vi "FeedbackDecode_FPPNS2NIP.vi"(5 "NIPTime":dbl=37572.0, 6 "EncodeClust":T2={"ParamsTable"=[], "Sel"=[], "Stim"=FALSE, "StimMode"=enum."Off", "StimStep"=[enum."1uA", enum."1uA", enum."Off"], "Jitter"=FALSE, "Pulse"=FALSE, "BFreq"=0.0, "BAmp"=0.0, "UEAArray"=[], "AdjClust"={"Add"=FALSE, "Sub"=FALSE, "Val"=[1.0, 100.0, 0.2, 500.0, 0.0], "B"=[FALSE, FALSE, FALSE, FALSE, FALSE], "Inc+"=["x+1", "x+10", "x+0.1", "x+10", "x+10"], "Set"=FALSE, "LoadTable"=FALSE, "SaveTable"=FALSE, "ClearTable"=FALSE, "DeleteSel"=FALSE, "Inc-"=["x-1", "x-10", "x-0.1", "x-10", "x-10"]}, "PresetTable"=[], "SelPreset"=[], "SortClust"={"Region"=FALSE, "Receptor"=FALSE, "Electrode"=FALSE, "Min Amp"=FALSE, "Max Amp"=FALSE, "Min Freq"=FALSE, "Max Freq"=FALSE, "Duration"=FALSE}, "SelSort"={"Sel"=FALSE}, "PresetClust"={"Load"=FALSE, "Clear"=FALSE, "Save"=FALSE, "Del"=FALSE}, "RespClust"={"RespType"=enum."Sensor Map", "OpenResp"=FALSE}, "AmpLimit"=0.0, "FreqLimit"=0.0, "DurLimit"=0.0, "Wait Period"=0.0, "Train Period"=0.0} {"Train Period" min=0.0 max=100.0 step=0.1; "Wait Period" min=0.0 max=100.0 step=0.1; "DurLimit" min=0.0 max=1.0 step=0.01; "FreqLimit" min=0.0 max=500.0 step=1.0; "AmpLimit" min=0.0 max=100.0 step=1.0; "BAmp" min=0.0 max=100.0 step=1.0; "BFreq" min=0.0 max=100.0 step=1.0}, 7 "LoopCnt":dbl=37572.0, 8 "DecodeClust":T3={"TrainParams"={"Lag"=0.0, "KernelWidth"=0.3, "TargRad"=0.15}, "Kinematics"={"Thumb"=0.0, "Index"=0.0, "Middle"=0.0, "Ring"=0.0, "Little"=0.0, "ThumbInt"=0.0, "IndexInt"=0.0, "RingInt"=0.0, "LittleInt"=0.0, "Wrist"=0.0, "WristYaw"=0.0, "WristRoll"=0.0}, "CtrlButtons"={"AcqTraining"=FALSE, "ApplyBaseline"=FALSE, "ApplyTraining"=FALSE, "LoadTrainFile"=FALSE, "CAR"=FALSE, "NIPSpikes"=FALSE, "AcqBaseline"=FALSE, "Stop"=FALSE, "ResetTrial"=FALSE, "CalDEKA"=FALSE, "HideSphrs"=FALSE, "StartTrials"=FALSE, "AutoPop"=FALSE, "ResetVRE"=FALSE, "StopVRE"=FALSE, "AcqCAR"=FALSE, "ConARD"=FALSE, "DEKARestart"=FALSE, "ConnDEKA"=FALSE}, "CompID"={"LV"={"Name"="PNILABVIEW", "IP"="155.100.90.215"}, "ML"={"Name"="PNIMATLAB", "IP"="155.100.91.231"}}, "KMvntClust"={"KGain"=[[1.0, 1.0, -1.0, 1.0], [1.0, 1.0, -1.0, 1.0], [1.0, 1.0, -1.0, 1.0], [1.0, 1.0, -1.0, 1.0], [1.0, 1.0, -1.0, 1.0], [1.0, 1.0, -1.0, 1.0], [1.0, 1.0, -1.0, 1.0], [1.0, 1.0, -1.0, 1.0], [1.0, 1.0, -1.0, 1.0], [1.0, 1.0, -1.0, 1.0], [1.0, 1.0, -1.0, 1.0], [1.0, 1.0, -1.0, 1.0]], "KMvnts"={"Thumb"=FALSE, "Index"=FALSE, "Middle"=FALSE, "Ring"=FALSE, "Little"=FALSE, "ThumbInt"=FALSE, "IndexInt"=FALSE, "RingInt"=FALSE, "LittleInt"=FALSE, "WristPitch"=FALSE, "WristYaw"=FALSE, "WristRoll"=FALSE}, "KThresh"=[[0.2, 0.2, -1.0, 1.0], [0.2, 0.2, -1.0, 1.0], [0.2, 0.2, -1.0, 1.0], [0.2, 0.2, -1.0, 1.0], [0.2, 0.2, -1.0, 1.0], [0.2, 0.2, -1.0, 1.0], [0.2, 0.2, -1.0, 1.0], [0.2, 0.2, -1.0, 1.0], [0.2, 0.2, -1.0, 1.0], [0.2, 0.2, -1.0, 1.0], [0.2, 0.2, -1.0, 1.0], [0.2, 0.2, -1.0, 1.0]], "CtrlMode"=[], "CtrlSpd"=[]}, "ClearUEA"=FALSE, "Targets"={"Thumb"=0.0, "Index"=0.0, "Middle"=0.0, "Ring"=0.0, "Little"=0.0, "ThumbInt"=0.0, "IndexInt"=0.0, "RingInt"=0.0, "LittleInt"=0.0, "Wrist"=0.0, "WristYaw"=0.0, "WristRoll"=0.0}, "KUEAArray"=[{"Boolean 1"=FALSE, "Boolean 2"=FALSE, "Boolean 3"=FALSE, "Boolean 4"=FALSE, "Boolean 5"=FALSE, "Boolean 6"=FALSE, "Boolean 7"=FALSE, "Boolean 8"=FALSE, "Boolean 9"=FALSE, "Boolean 10"=FALSE, "Boolean 11"=FALSE, "Boolean 12"=FALSE, "Boolean 13"=FALSE, "Boolean 14"=FALSE, "Boolean 15"=FALSE, "Boolean 16"=FALSE, "Boolean 17"=FALSE, "Boolean 18"=FALSE, "Boolean 19"=FALSE, "Boolean 20"=FALSE, "Boolean 21"=FALSE, "Boolean 22"=FALSE, "Boolean 23"=FALSE, "Boolean 24"=FALSE, "Boolean 25"=FALSE, "Boolean 26"=FALSE, "Boolean 27"=FALSE, "Boolean 28"=FALSE, "Boolean 29"=FALSE, "Boolean 30"=FALSE, "Boolean 31"=FALSE, "Boolean 32"=FALSE, "Boolean 33"=FALSE, "Boolean 34"=FALSE, "Boolean 35"=FALSE, "Boolean 36"=FALSE, "Boolean 37"=FALSE, "Boolean 38"=FALSE, "Boolean 39"=FALSE, "Boolean 40"=FALSE, "Boolean 41"=FALSE, "Boolean 42"=FALSE, "Boolean 43"=FALSE, "Boolean 44"=FALSE, "Boolean 45"=FALSE, "Boolean 46"=FALSE, "Boolean 47"=FALSE, "Boolean 48"=FALSE, "Boolean 49"=FALSE, "Boolean 50"=FALSE, "Boolean 51"=FALSE, "Boolean 52"=FALSE, "Boolean 53"=FALSE, "Boolean 54"=FALSE, "Boolean 55"=FALSE, "Boolean 56"=FALSE, "Boolean 57"=FALSE, "Boolean 58"=FALSE, "Boolean 59"=FALSE, "Boolean 60"=FALSE, "Boolean 61"=FALSE, "Boolean 62"=FALSE, "Boolean 63"=FALSE, "Boolean 64"=FALSE, "Boolean 65"=FALSE, "Boolean 66"=FALSE, "Boolean 67"=FALSE, "Boolean 68"=FALSE, "Boolean 69"=FALSE, "Boolean 70"=FALSE, "Boolean 71"=FALSE, "Boolean 72"=FALSE, "Boolean 73"=FALSE, "Boolean 74"=FALSE, "Boolean 75"=FALSE, "Boolean 76"=FALSE, "Boolean 77"=FALSE, "Boolean 78"=FALSE, "Boolean 79"=FALSE, "Boolean 80"=FALSE, "Boolean 81"=FALSE, "Boolean 82"=FALSE, "Boolean 83"=FALSE, "Boolean 84"=FALSE, "Boolean 85"=FALSE, "Boolean 86"=FALSE, "Boolean 87"=FALSE, "Boolean 88"=FALSE, "Boolean 89"=FALSE, "Boolean 90"=FALSE, "Boolean 91"=FALSE, "Boolean 92"=FALSE, "Boolean 93"=FALSE, "Boolean 94"=FALSE, "Boolean 95"=FALSE, "Boolean 96"=FALSE, "Boolean 97"=FALSE, "Boolean 98"=FALSE, "Boolean 99"=FALSE, "Boolean 100"=FALSE}, {"Boolean 1"=FALSE, "Boolean 2"=FALSE, "Boolean 3"=FALSE, "Boolean 4"=FALSE, "Boolean 5"=FALSE, "Boolean 6"=FALSE, "Boolean 7"=FALSE, "Boolean 8"=FALSE, "Boolean 9"=FALSE, "Boolean 10"=FALSE, "Boolean 11"=FALSE, "Boolean 12"=FALSE, "Boolean 13"=FALSE, "Boolean 14"=FALSE, "Boolean 15"=FALSE, "Boolean 16"=FALSE, "Boolean 17"=FALSE, "Boolean 18"=FALSE, "Boolean 19"=FALSE, "Boolean 20"=FALSE, "Boolean 21"=FALSE, "Boolean 22"=FALSE, "Boolean 23"=FALSE, "Boolean 24"=FALSE, "Boolean 25"=FALSE, "Boolean 26"=FALSE, "Boolean 27"=FALSE, "Boolean 28"=FALSE, "Boolean 29"=FALSE, "Boolean 30"=FALSE, "Boolean 31"=FALSE, "Boolean 32"=FALSE, "Boolean 33"=FALSE, "Boolean 34"=FALSE, "Boolean 35"=FALSE, "Boolean 36"=FALSE, "Boolean 37"=FALSE, "Boolean 38"=FALSE, "Boolean 39"=FALSE, "Boolean 40"=FALSE, "Boolean 41"=FALSE, "Boolean 42"=FALSE, "Boolean 43"=FALSE, "Boolean 44"=FALSE, "Boolean 45"=FALSE, "Boolean 46"=FALSE, "Boolean 47"=FALSE, "Boolean 48"=FALSE, "Boolean 49"=FALSE, "Boolean 50"=FALSE, "Boolean 51"=FALSE, "Boolean 52"=FALSE, "Boolean 53"=FALSE, "Boolean 54"=FALSE, "Boolean 55"=FALSE, "Boolean 56"=FALSE, "Boolean 57"=FALSE, "Boolean 58"=FALSE, "Boolean 59"=FALSE, "Boolean 60"=FALSE, "Boolean 61"=FALSE, "Boolean 62"=FALSE, "Boolean 63"=FALSE, "Boolean 64"=FALSE, "Boolean 65"=FALSE, "Boolean 66"=FALSE, "Boolean 67"=FALSE, "Boolean 68"=FALSE, "Boolean 69"=FALSE, "Boolean 70"=FALSE, "Boolean 71"=FALSE, "Boolean 72"=FALSE, "Boolean 73"=FALSE, "Boolean 74"=FALSE, "Boolean 75"=FALSE, "Boolean 76"=FALSE, "Boolean 77"=FALSE, "Boolean 78"=FALSE, "Boolean 79"=FALSE, "Boolean 80"=FALSE, "Boolean 81"=FALSE, "Boolean 82"=FALSE, "Boolean 83"=FALSE, "Boolean 84"=FALSE, "Boolean 85"=FALSE, "Boolean 86"=FALSE, "Boolean 87"=FALSE, "Boolean 88"=FALSE, "Boolean 89"=FALSE, "Boolean 90"=FALSE, "Boolean 91"=FALSE, "Boolean 92"=FALSE, "Boolean 93"=FALSE, "Boolean 94"=FALSE, "Boolean 95"=FALSE, "Boolean 96"=FALSE, "Boolean 97"=FALSE, "Boolean 98"=FALSE, "Boolean 99"=FALSE, "Boolean 100"=FALSE}], "ReTrain"=FALSE, "TargDist"=[0.0, 0.0, 0.0, 0.0, 0.0, 0.0], "State"=enum."Initialize", "KalmanType"=enum."Standard", "EventStr"="", "SelElect"=1.0, "KinSrc"=enum."Training", "HoverElect"=0.0, "RasterWin"=1.0, "WfCnt"=15.0, "ClearWfs"=FALSE, "ApplyThresh"=FALSE, "ThreshVal"=-5.0, "ThreshMode"=enum."RMS Single", "DataFolder"="00000000-000000", "ClearEMG"=FALSE, "KEMGClust"={"Boolean 92"=FALSE, "Boolean 82"=FALSE, "Boolean 72"=FALSE, "Boolean 62"=FALSE, "Boolean 52"=FALSE, "Boolean 42"=FALSE, "Boolean 32"=FALSE, "Boolean 22"=FALSE, "Boolean 12"=FALSE, "Boolean 2"=FALSE, "Boolean 93"=FALSE, "Boolean 83"=FALSE, "Boolean 73"=FALSE, "Boolean 63"=FALSE, "Boolean 53"=FALSE, "Boolean 43"=FALSE, "Boolean 33"=FALSE, "Boolean 23"=FALSE, "Boolean 13"=FALSE, "Boolean 3"=FALSE, "Boolean 94"=FALSE, "Boolean 84"=FALSE, "Boolean 74"=FALSE, "Boolean 64"=FALSE, "Boolean 54"=FALSE, "Boolean 44"=FALSE, "Boolean 34"=FALSE, "Boolean 24"=FALSE, "Boolean 14"=FALSE, "Boolean 4"=FALSE, "Boolean 95"=FALSE, "Boolean 85"=FALSE, "Boolean 75"=FALSE, "Boolean 65"=FALSE, "Boolean 55"=FALSE, "Boolean 45"=FALSE, "Boolean 35"=FALSE, "Boolean 25"=FALSE, "Boolean 15"=FALSE, "Boolean 5"=FALSE, "Boolean 96"=FALSE, "Boolean 86"=FALSE, "Boolean 76"=FALSE, "Boolean 66"=FALSE, "Boolean 56"=FALSE, "Boolean 46"=FALSE, "Boolean 36"=FALSE, "Boolean 26"=FALSE, "Boolean 16"=FALSE, "Boolean 6"=FALSE, "Boolean 97"=FALSE, "Boolean 87"=FALSE, "Boolean 77"=FALSE, "Boolean 67"=FALSE, "Boolean 57"=FALSE, "Boolean 47"=FALSE, "Boolean 37"=FALSE, "Boolean 27"=FALSE, "Boolean 17"=FALSE, "Boolean 7"=FALSE, "Boolean 98"=FALSE, "Boolean 88"=FALSE, "Boolean 78"=FALSE, "Boolean 68"=FALSE, "Boolean 58"=FALSE, "Boolean 48"=FALSE, "Boolean 38"=FALSE, "Boolean 28"=FALSE, "Boolean 18"=FALSE, "Boolean 8"=FALSE, "Boolean 99"=FALSE, "Boolean 89"=FALSE, "Boolean 79"=FALSE, "Boolean 69"=FALSE, "Boolean 59"=FALSE, "Boolean 49"=FALSE, "Boolean 39"=FALSE, "Boolean 29"=FALSE, "Boolean 19"=FALSE, "Boolean 9"=FALSE}, "EvntFlag"=FALSE, "FillUEA"=FALSE, "FillEMG"=FALSE, "FillMvnts"=FALSE, "BadUEAElects"=[], "KEMGExtra"=[], "AllPairs"=FALSE, "AutoThresh"=0.4, "BadEMGChans"=[], "LinkedDOF"="{}", "AutoPopType"=enum."Standard", "CARType"=enum."Standard", "*Map"=enum."pNeural/pEMG", "GainFill"=1.0, "ThreshFill"=1.0, "TestType"=enum."MSMS", "Outcome"=enum."---", "TrialCnt"=[], "ClearTrials"=FALSE, "Log10"=FALSE, "KDFFile"="{}", "LimitExt"=FALSE, "*Prosthesis"=enum."MaleLeft", "StartML"=FALSE, "StartMLAux"=FALSE, "StartRec"=FALSE, "DynaThr"=FALSE, "ModeFill"=enum."Position", "SpdFill"=1.0, "DEKAMode"=enum."Velocity", "FreeParam"=0.4, "GoalNoise"=0.4, "Load NN"=FALSE, "ExportTrain"=FALSE, "NumComp"=enum."2 Computers", "DataDir"="00000000-000000", "BuildDir"="00000000-000000", "LatchingFilter"=FALSE, "Trigger"=FALSE, "StartARD"=FALSE, "StartTaska"=FALSE, "StartTaskaSens"=FALSE} {"SpdFill" min=0.0 max=10.0 step=0.1; "RasterWin" min=1.0 max=30.0 step=1.0; "ThreshFill" min=0.0 max=10.0 step=0.01; "GainFill" min=0.0 max=10.0 step=0.1; "AutoThresh" min=0.0 max=1.0; "Targets"."LittleInt" min=0.0 max=1.0 step=0.01; "Targets"."WristRoll" min=0.0 max=1.0 step=0.01; "Targets"."WristYaw" min=0.0 max=1.0 step=0.01; "Targets"."Wrist" min=0.0 max=1.0 step=0.01; "Targets"."Little" min=0.0 max=1.0 step=0.01; "Targets"."Thumb" min=0.0 max=1.0 step=0.01; "Targets"."RingInt" min=0.0 max=1.0 step=0.01; "Targets"."IndexInt" min=0.0 max=1.0 step=0.01; "Targets"."ThumbInt" min=0.0 max=1.0 step=0.01; "Targets"."Ring" min=0.0 max=1.0 step=0.01; "Targets"."Middle" min=0.0 max=1.0 step=0.01; "Targets"."Index" min=0.0 max=1.0 step=0.01; "KMvntClust"."CtrlSpd" min=0 max=10; "KMvntClust"."KThresh" min=0 max=1; "KMvntClust"."KGain" min=0; "Kinematics"."LittleInt" min=0.0 max=1.0 step=0.01; "Kinematics"."WristRoll" min=0.0 max=1.0 step=0.01; "Kinematics"."WristYaw" min=0.0 max=1.0 step=0.01; "Kinematics"."Wrist" min=0.0 max=1.0 step=0.01; "Kinematics"."Little" min=0.0 max=1.0 step=0.01; "Kinematics"."Thumb" min=0.0 max=1.0 step=0.01; "Kinematics"."RingInt" min=0.0 max=1.0 step=0.01; "Kinematics"."IndexInt" min=0.0 max=1.0 step=0.01; "Kinematics"."ThumbInt" min=0.0 max=1.0 step=0.01; "Kinematics"."Ring" min=0.0 max=1.0 step=0.01; "Kinematics"."Middle" min=0.0 max=1.0 step=0.01; "Kinematics"."Index" min=0.0 max=1.0 step=0.01; "TrainParams"."TargRad" step=0.05 format="%#.2g"; "TrainParams"."KernelWidth" step=0.05 format="%#.2g"}, 9 "TrialTiming":T4={"Dur"={"ASD"=1000, "ARD"=1000, "ART"=3000, "ETD"=2000}, "Rnd"={"ASDR"=0, "ARDR"=0, "ARTR"=0, "ETDR"=0}, "Act"={"ASDA"=1000, "ARDA"=1000, "ARTA"=3000, "ETDA"=2000}} caption="Trial Timing", 10 "TargParams":cluster{"Gain":dbl, "Radius":dbl, "Acc":dbl}={"Gain"=1.0, "Radius"=0.12, "Acc"=0.8} caption="Target Parameters" {"Acc" min=0.0 max=1.0 step=0.01; "Radius" min=0.0 max=1.0 step=0.01; "Gain" min=-1.0 max=1.0 step=0.01}, 11 "MvntClust":T1={"MvntMat"=[], "MvntName"="", "Tracking"=enum."False", "Radius"=0.15} {"Radius" min=0.0 max=1.0 step=0.01}) -> (1 "TrialParams":string)   [LabVIEW 2020]
uses:
  FeedbackDecode_DecodeClust.ctl
  FeedbackDecode_EncodeClust.ctl
  FeedbackDecode_VariablesToString_Scalar.vi
  FeedbackDecode_VariablesToString_Array.vi
  FeedbackDecode_VariablesToString_String.vi
panel:
  # "Thumb"
  # "Index"
  # "Middle"
  # "Ring"
  # "Little"
  # "ThumbInt"
  # "IndexInt"
  # "RingInt"
  # "LittleInt"
  # "WristPitch"
  # "WristYaw"
  # "WristRoll"
  # "Amp"
  # "Del"
  # "Rise"
  # "Hold"
  # "Value"
  # "Inc-"
  # "Inc+"
  # "Min Amp"
  # "Max Amp"
  # "Min Freq"
  # "Max Freq"
  # "Duration"
  # "G"
  # "T"
  # "Mode"
  # "S"
  # "Negative lag shifts feature variables left (earlier)"
  # "{[1,2,4];[5,3];[6,7,8]}"
  # "Select before apply training"
  # "1"
  # "2"
  # "3"
  # "4"
  # "5"
  # "6"
  # "7"
  # "8"
  # "1"
  # "2"
  # "3"
  # "4"
  # "1-2"
  # "1-3"
  # "1-4"
  # "2-3"
  # "2-4"
  # "3-4"
  # "DOF"
  # "Gain (F/E)"
  # "Thresh (F/E)"
  # "Mode"
  # "Spd"
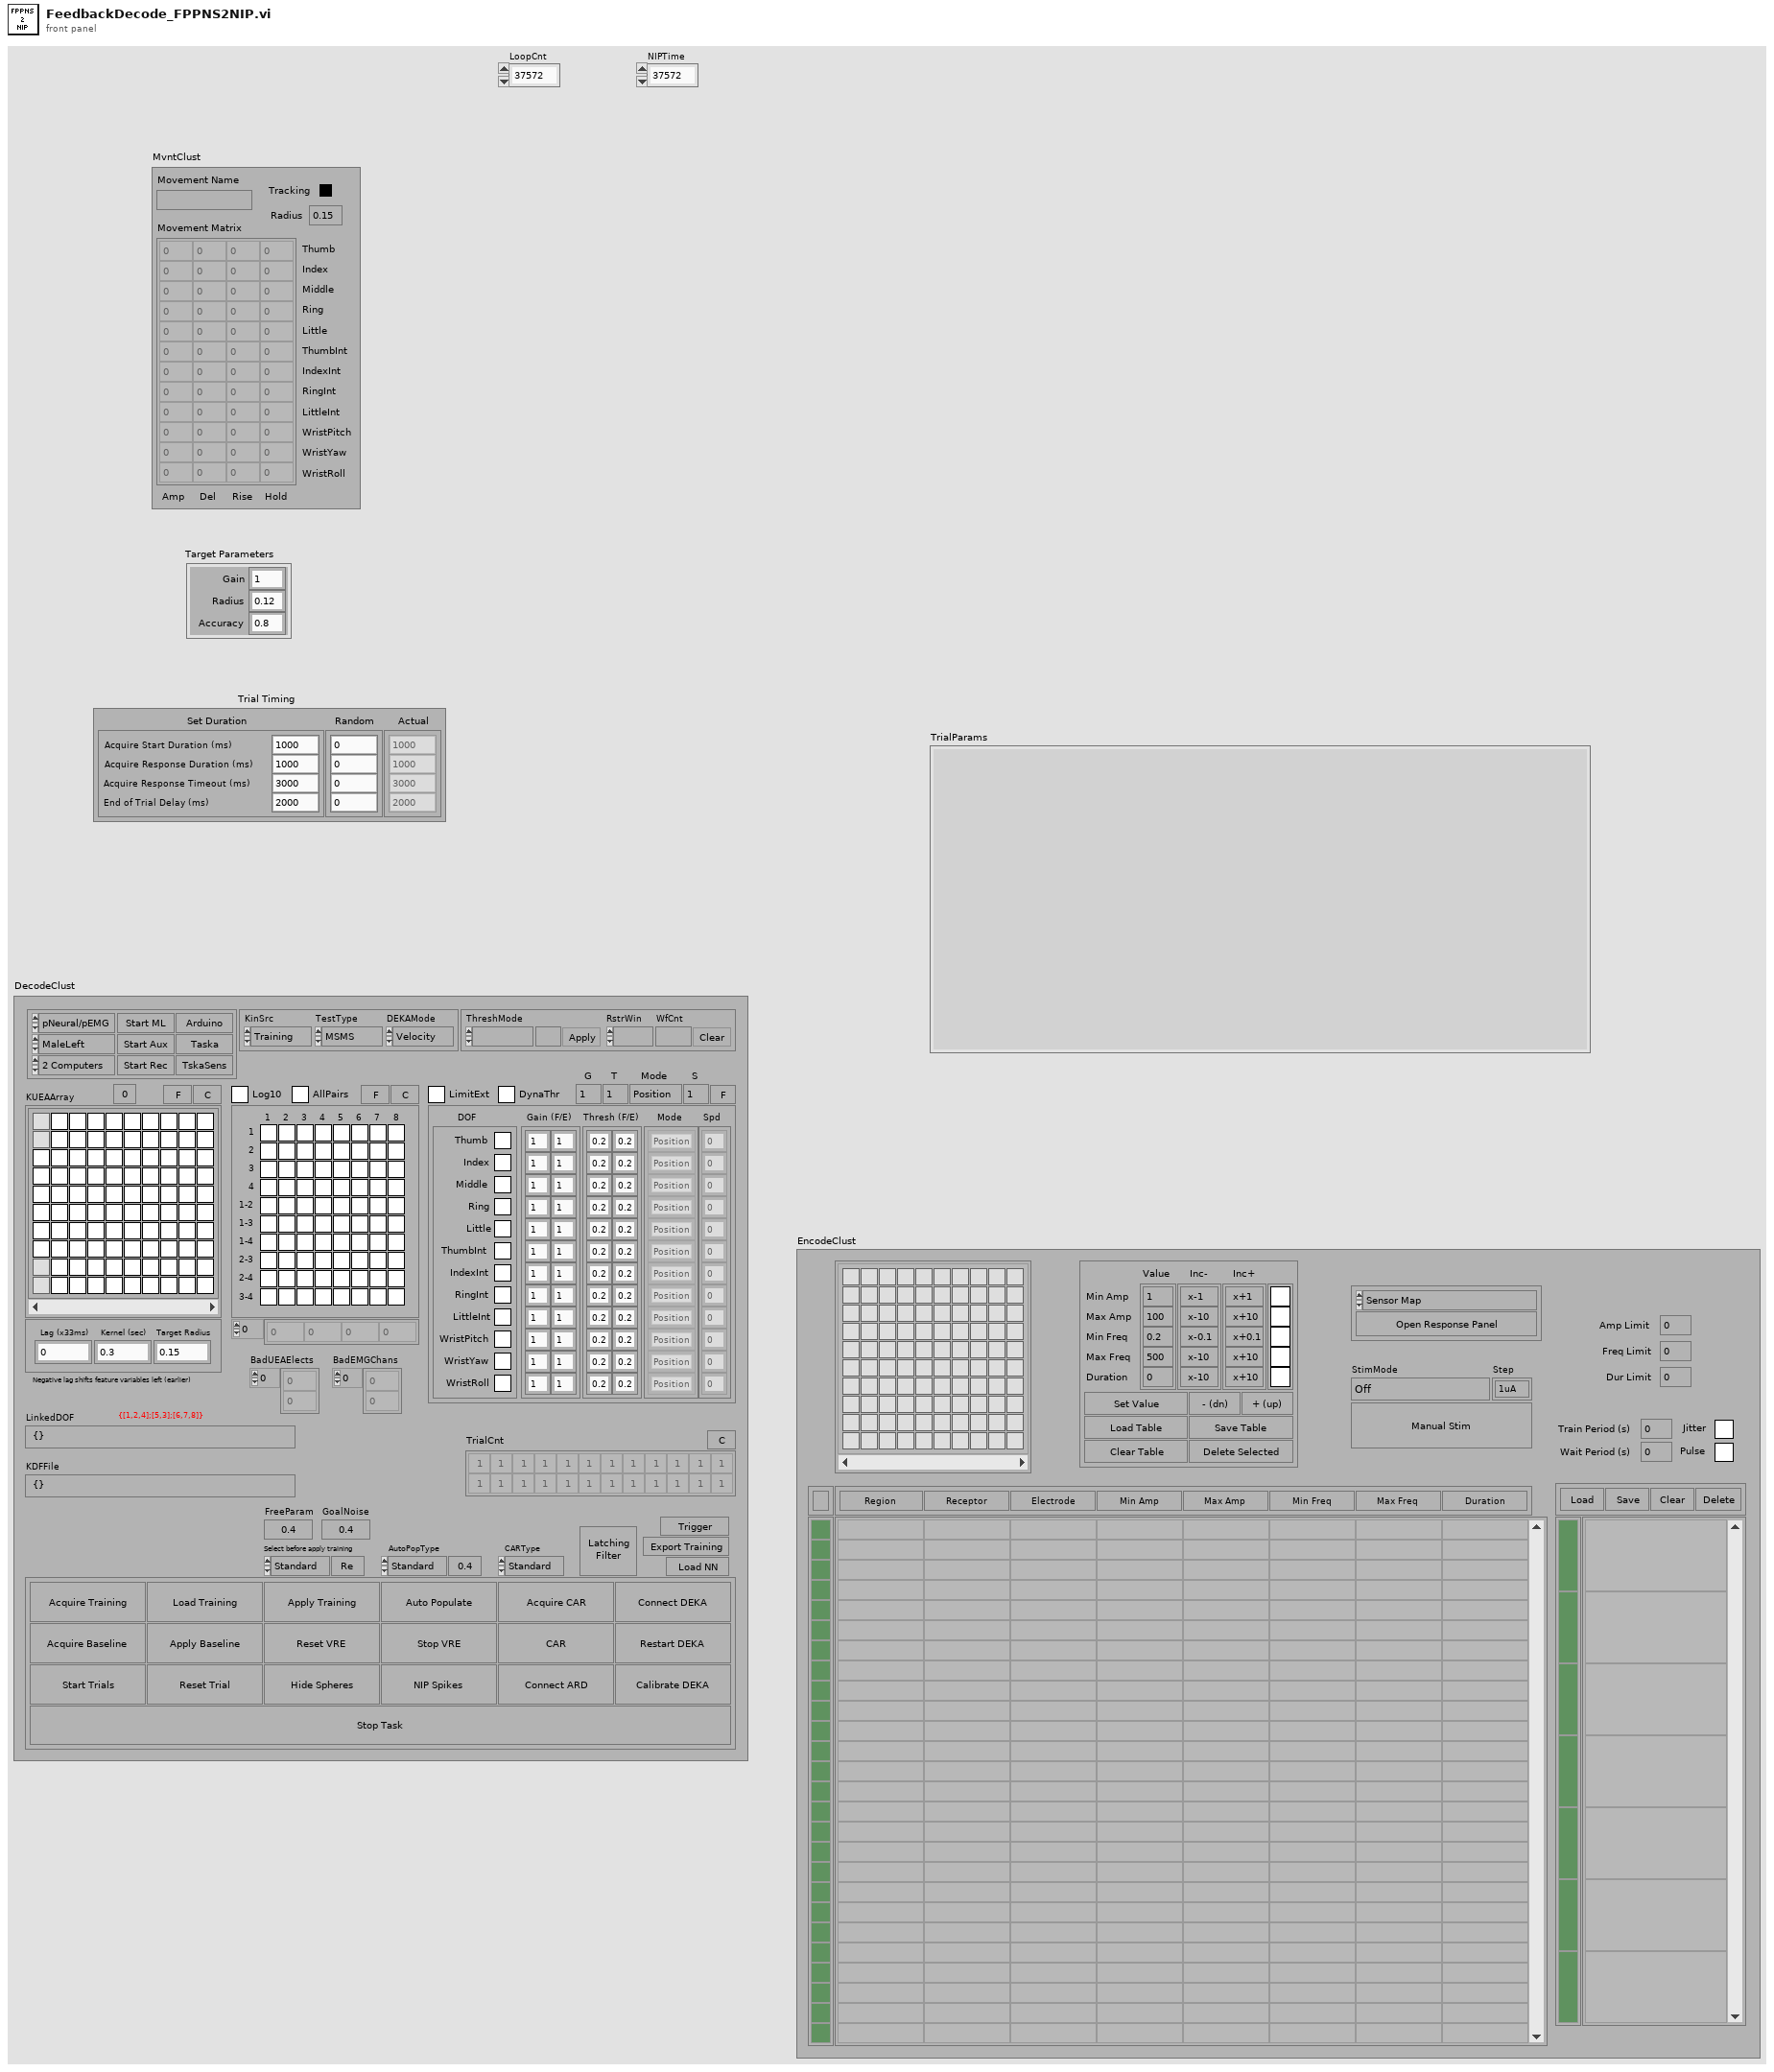
[diagram p1: front panel]
types:
  T1 = cluster{"MvntMat":dbl[][], "MvntName":string, "Tracking":enum8{"False", "True", "Mixed"}, "Radius":dbl}
  T2 = typedef "FeedbackDecode_EncodeClust.ctl" = cluster{"ParamsTable":string[][], "Sel":bool[], "Stim":bool, "StimMode":enum16{"Off", "Manual", "MSMS", "VRE", "3DHand", "DEKA", "Analog(DEKA)"}, "StimStep":enum16{"Off", "1uA", "2uA", "5uA", "10uA", "20uA", "30uA"}[], "Jitter":bool, "Pulse":bool, "BFreq":dbl, "BAmp":dbl, "UEAArray":cluster{"Boolean 1":bool, "Boolean 2":bool, "Boolean 3":bool, "Boolean 4":bool, "Boolean 5":bool, "Boolean 6":bool, "Boolean 7":bool, "Boolean 8":bool, "Boolean 9":bool, "Boolean 10":bool, "Boolean 11":bool, "Boolean 12":bool, "Boolean 13":bool, "Boolean 14":bool, "Boolean 15":bool, "Boolean 16":bool, "Boolean 17":bool, "Boolean 18":bool, "Boolean 19":bool, "Boolean 20":bool, "Boolean 21":bool, "Boolean 22":bool, "Boolean 23":bool, "Boolean 24":bool, "Boolean 25":bool, "Boolean 26":bool, "Boolean 27":bool, "Boolean 28":bool, "Boolean 29":bool, "Boolean 30":bool, "Boolean 31":bool, "Boolean 32":bool, "Boolean 33":bool, "Boolean 34":bool, "Boolean 35":bool, "Boolean 36":bool, "Boolean 37":bool, "Boolean 38":bool, "Boolean 39":bool, "Boolean 40":bool, "Boolean 41":bool, "Boolean 42":bool, "Boolean 43":bool, "Boolean 44":bool, "Boolean 45":bool, "Boolean 46":bool, "Boolean 47":bool, "Boolean 48":bool, "Boolean 49":bool, "Boolean 50":bool, "Boolean 51":bool, "Boolean 52":bool, "Boolean 53":bool, "Boolean 54":bool, "Boolean 55":bool, "Boolean 56":bool, "Boolean 57":bool, "Boolean 58":bool, "Boolean 59":bool, "Boolean 60":bool, "Boolean 61":bool, "Boolean 62":bool, "Boolean 63":bool, "Boolean 64":bool, "Boolean 65":bool, "Boolean 66":bool, "Boolean 67":bool, "Boolean 68":bool, "Boolean 69":bool, "Boolean 70":bool, "Boolean 71":bool, "Boolean 72":bool, "Boolean 73":bool, "Boolean 74":bool, "Boolean 75":bool, "Boolean 76":bool, "Boolean 77":bool, "Boolean 78":bool, "Boolean 79":bool, "Boolean 80":bool, "Boolean 81":bool, "Boolean 82":bool, "Boolean 83":bool, "Boolean 84":bool, "Boolean 85":bool, "Boolean 86":bool, "Boolean 87":bool, "Boolean 88":bool, "Boolean 89":bool, "Boolean 90":bool, "Boolean 91":bool, "Boolean 92":bool, "Boolean 93":bool, "Boolean 94":bool, "Boolean 95":bool, "Boolean 96":bool, "Boolean 97":bool, "Boolean 98":bool, "Boolean 99":bool, "Boolean 100":bool}[], "AdjClust":cluster{"Add":bool, "Sub":bool, "Val":dbl[], "B":bool[], "Inc+":string[], "Set":bool, "LoadTable":bool, "SaveTable":bool, "ClearTable":bool, "DeleteSel":bool, "Inc-":string[]}, "PresetTable":string[][], "SelPreset":bool[], "SortClust":cluster{"Region":bool, "Receptor":bool, "Electrode":bool, "Min Amp":bool, "Max Amp":bool, "Min Freq":bool, "Max Freq":bool, "Duration":bool}, "SelSort":cluster{"Sel":bool}, "PresetClust":cluster{"Load":bool, "Clear":bool, "Save":bool, "Del":bool}, "RespClust":cluster{"RespType":enum16{"Sensor Map", "Full Map"}, "OpenResp":bool}, "AmpLimit":dbl, "FreqLimit":dbl, "DurLimit":dbl, "Wait Period":dbl, "Train Period":dbl}
  T3 = typedef "FeedbackDecode_DecodeClust.ctl" = cluster{"TrainParams":cluster{"Lag":dbl, "KernelWidth":dbl, "TargRad":dbl}, "Kinematics":cluster{"Thumb":dbl, "Index":dbl, "Middle":dbl, "Ring":dbl, "Little":dbl, "ThumbInt":dbl, "IndexInt":dbl, "RingInt":dbl, "LittleInt":dbl, "Wrist":dbl, "WristYaw":dbl, "WristRoll":dbl}, "CtrlButtons":cluster{"AcqTraining":bool, "ApplyBaseline":bool, "ApplyTraining":bool, "LoadTrainFile":bool, "CAR":bool, "NIPSpikes":bool, "AcqBaseline":bool, "Stop":bool, "ResetTrial":bool, "CalDEKA":bool, "HideSphrs":bool, "StartTrials":bool, "AutoPop":bool, "ResetVRE":bool, "StopVRE":bool, "AcqCAR":bool, "ConARD":bool, "DEKARestart":bool, "ConnDEKA":bool}, "CompID":cluster{"LV":cluster{"Name":string, "IP":string}, "ML":cluster{"Name":string, "IP":string}}, "KMvntClust":cluster{"KGain":sgl[][], "KMvnts":cluster{"Thumb":bool, "Index":bool, "Middle":bool, "Ring":bool, "Little":bool, "ThumbInt":bool, "IndexInt":bool, "RingInt":bool, "LittleInt":bool, "WristPitch":bool, "WristYaw":bool, "WristRoll":bool}, "KThresh":sgl[][], "CtrlMode":enum16{"Position", "Latching", "Leaky", "Velocity"}[], "CtrlSpd":sgl[]}, "ClearUEA":bool, "Targets":cluster{"Thumb":dbl, "Index":dbl, "Middle":dbl, "Ring":dbl, "Little":dbl, "ThumbInt":dbl, "IndexInt":dbl, "RingInt":dbl, "LittleInt":dbl, "Wrist":dbl, "WristYaw":dbl, "WristRoll":dbl}, "KUEAArray":cluster{"Boolean 1":bool, "Boolean 2":bool, "Boolean 3":bool, "Boolean 4":bool, "Boolean 5":bool, "Boolean 6":bool, "Boolean 7":bool, "Boolean 8":bool, "Boolean 9":bool, "Boolean 10":bool, "Boolean 11":bool, "Boolean 12":bool, "Boolean 13":bool, "Boolean 14":bool, "Boolean 15":bool, "Boolean 16":bool, "Boolean 17":bool, "Boolean 18":bool, "Boolean 19":bool, "Boolean 20":bool, "Boolean 21":bool, "Boolean 22":bool, "Boolean 23":bool, "Boolean 24":bool, "Boolean 25":bool, "Boolean 26":bool, "Boolean 27":bool, "Boolean 28":bool, "Boolean 29":bool, "Boolean 30":bool, "Boolean 31":bool, "Boolean 32":bool, "Boolean 33":bool, "Boolean 34":bool, "Boolean 35":bool, "Boolean 36":bool, "Boolean 37":bool, "Boolean 38":bool, "Boolean 39":bool, "Boolean 40":bool, "Boolean 41":bool, "Boolean 42":bool, "Boolean 43":bool, "Boolean 44":bool, "Boolean 45":bool, "Boolean 46":bool, "Boolean 47":bool, "Boolean 48":bool, "Boolean 49":bool, "Boolean 50":bool, "Boolean 51":bool, "Boolean 52":bool, "Boolean 53":bool, "Boolean 54":bool, "Boolean 55":bool, "Boolean 56":bool, "Boolean 57":bool, "Boolean 58":bool, "Boolean 59":bool, "Boolean 60":bool, "Boolean 61":bool, "Boolean 62":bool, "Boolean 63":bool, "Boolean 64":bool, "Boolean 65":bool, "Boolean 66":bool, "Boolean 67":bool, "Boolean 68":bool, "Boolean 69":bool, "Boolean 70":bool, "Boolean 71":bool, "Boolean 72":bool, "Boolean 73":bool, "Boolean 74":bool, "Boolean 75":bool, "Boolean 76":bool, "Boolean 77":bool, "Boolean 78":bool, "Boolean 79":bool, "Boolean 80":bool, "Boolean 81":bool, "Boolean 82":bool, "Boolean 83":bool, "Boolean 84":bool, "Boolean 85":bool, "Boolean 86":bool, "Boolean 87":bool, "Boolean 88":bool, "Boolean 89":bool, "Boolean 90":bool, "Boolean 91":bool, "Boolean 92":bool, "Boolean 93":bool, "Boolean 94":bool, "Boolean 95":bool, "Boolean 96":bool, "Boolean 97":bool, "Boolean 98":bool, "Boolean 99":bool, "Boolean 100":bool}[], "ReTrain":bool, "TargDist":dbl[], "State":enum16{"Initialize", "Acquire Start", "Acquire Response", "Finalize"}, "KalmanType":enum16{"Standard", "Mean", "Refit", "LinSVReg", "NonLinSVReg", "PCA", "DWPRR", "AdaptKF", "NN", "NN_python", "AdaptKF2", "KF_Short_Goal"}, "EventStr":string, "SelElect":dbl, "KinSrc":enum16{"Off", "Training", "Decode", "COB", "LEAP"}, "HoverElect":dbl, "RasterWin":dbl, "WfCnt":dbl, "ClearWfs":bool, "ApplyThresh":bool, "ThreshVal":dbl, "ThreshMode":enum16{"RMS Single", "RMS All", "RMS Auto", "Volt Single", "Volt All"}, "DataFolder":string, "ClearEMG":bool, "KEMGClust":cluster{"Boolean 92":bool, "Boolean 82":bool, "Boolean 72":bool, "Boolean 62":bool, "Boolean 52":bool, "Boolean 42":bool, "Boolean 32":bool, "Boolean 22":bool, "Boolean 12":bool, "Boolean 2":bool, "Boolean 93":bool, "Boolean 83":bool, "Boolean 73":bool, "Boolean 63":bool, "Boolean 53":bool, "Boolean 43":bool, "Boolean 33":bool, "Boolean 23":bool, "Boolean 13":bool, "Boolean 3":bool, "Boolean 94":bool, "Boolean 84":bool, "Boolean 74":bool, "Boolean 64":bool, "Boolean 54":bool, "Boolean 44":bool, "Boolean 34":bool, "Boolean 24":bool, "Boolean 14":bool, "Boolean 4":bool, "Boolean 95":bool, "Boolean 85":bool, "Boolean 75":bool, "Boolean 65":bool, "Boolean 55":bool, "Boolean 45":bool, "Boolean 35":bool, "Boolean 25":bool, "Boolean 15":bool, "Boolean 5":bool, "Boolean 96":bool, "Boolean 86":bool, "Boolean 76":bool, "Boolean 66":bool, "Boolean 56":bool, "Boolean 46":bool, "Boolean 36":bool, "Boolean 26":bool, "Boolean 16":bool, "Boolean 6":bool, "Boolean 97":bool, "Boolean 87":bool, "Boolean 77":bool, "Boolean 67":bool, "Boolean 57":bool, "Boolean 47":bool, "Boolean 37":bool, "Boolean 27":bool, "Boolean 17":bool, "Boolean 7":bool, "Boolean 98":bool, "Boolean 88":bool, "Boolean 78":bool, "Boolean 68":bool, "Boolean 58":bool, "Boolean 48":bool, "Boolean 38":bool, "Boolean 28":bool, "Boolean 18":bool, "Boolean 8":bool, "Boolean 99":bool, "Boolean 89":bool, "Boolean 79":bool, "Boolean 69":bool, "Boolean 59":bool, "Boolean 49":bool, "Boolean 39":bool, "Boolean 29":bool, "Boolean 19":bool, "Boolean 9":bool}, "EvntFlag":bool, "FillUEA":bool, "FillEMG":bool, "FillMvnts":bool, "BadUEAElects":dbl[], "KEMGExtra":dbl[], "AllPairs":bool, "AutoThresh":dbl, "BadEMGChans":dbl[], "LinkedDOF":string, "AutoPopType":enum16{"Standard", "Stepwise", "Gram"}, "CARType":enum16{"Standard", "NN"}, "*Map":enum16{"pNeural/pEMG", "pNeural/aEMG", "aNeural/pEMG", "aNeural/aEMG"}, "GainFill":dbl, "ThreshFill":dbl, "TestType":enum16{"MSMS", "Bakeoff11", "Bakeoff21", "Bakeoff31", "Bakeoff32", "Bakeoff32_Ball", "Bakeoff32_Checkers", "Bakeoff32_Pen", "FragileBlock"}, "Outcome":enum16{"---", "Success", "Failure"}, "TrialCnt":dbl[][], "ClearTrials":bool, "Log10":bool, "KDFFile":string, "LimitExt":bool, "*Prosthesis":enum16{"MaleRight", "MaleLeft"}, "StartML":bool, "StartMLAux":bool, "StartRec":bool, "DynaThr":bool, "ModeFill":enum16{"Position", "Latching", "Leaky", "Velocity"}, "SpdFill":dbl, "DEKAMode":enum16{"Velocity", "Position"}, "FreeParam":dbl, "GoalNoise":dbl, "Load NN":bool, "ExportTrain":bool, "NumComp":enum16{"1 Computer", "2 Computers"}, "DataDir":string, "BuildDir":string, "LatchingFilter":bool, "Trigger":bool, "StartARD":bool, "StartTaska":bool, "StartTaskaSens":bool}
  T4 = cluster{"Dur":cluster{"ASD":u16, "ARD":u16, "ART":u16, "ETD":u16}, "Rnd":cluster{"ASDR":u16, "ARDR":u16, "ARTR":u16, "ETDR":u16}, "Act":cluster{"ASDA":u16, "ARDA":u16, "ARTA":u16, "ETDA":u16}}
  T5 = enum16{"Off", "Training", "Decode", "COB", "LEAP"}
  T6 = enum16{"RMS Single", "RMS All", "RMS Auto", "Volt Single", "Volt All"}
  T7 = enum16{"Standard", "Mean", "Refit", "LinSVReg", "NonLinSVReg", "PCA", "DWPRR", "AdaptKF", "NN", "NN_python", "AdaptKF2", "KF_Short_Goal"}
  T8 = enum16{"pNeural/pEMG", "pNeural/aEMG", "aNeural/pEMG", "aNeural/aEMG"}
  T9 = enum16{"Position", "Latching", "Leaky", "Velocity"}[]
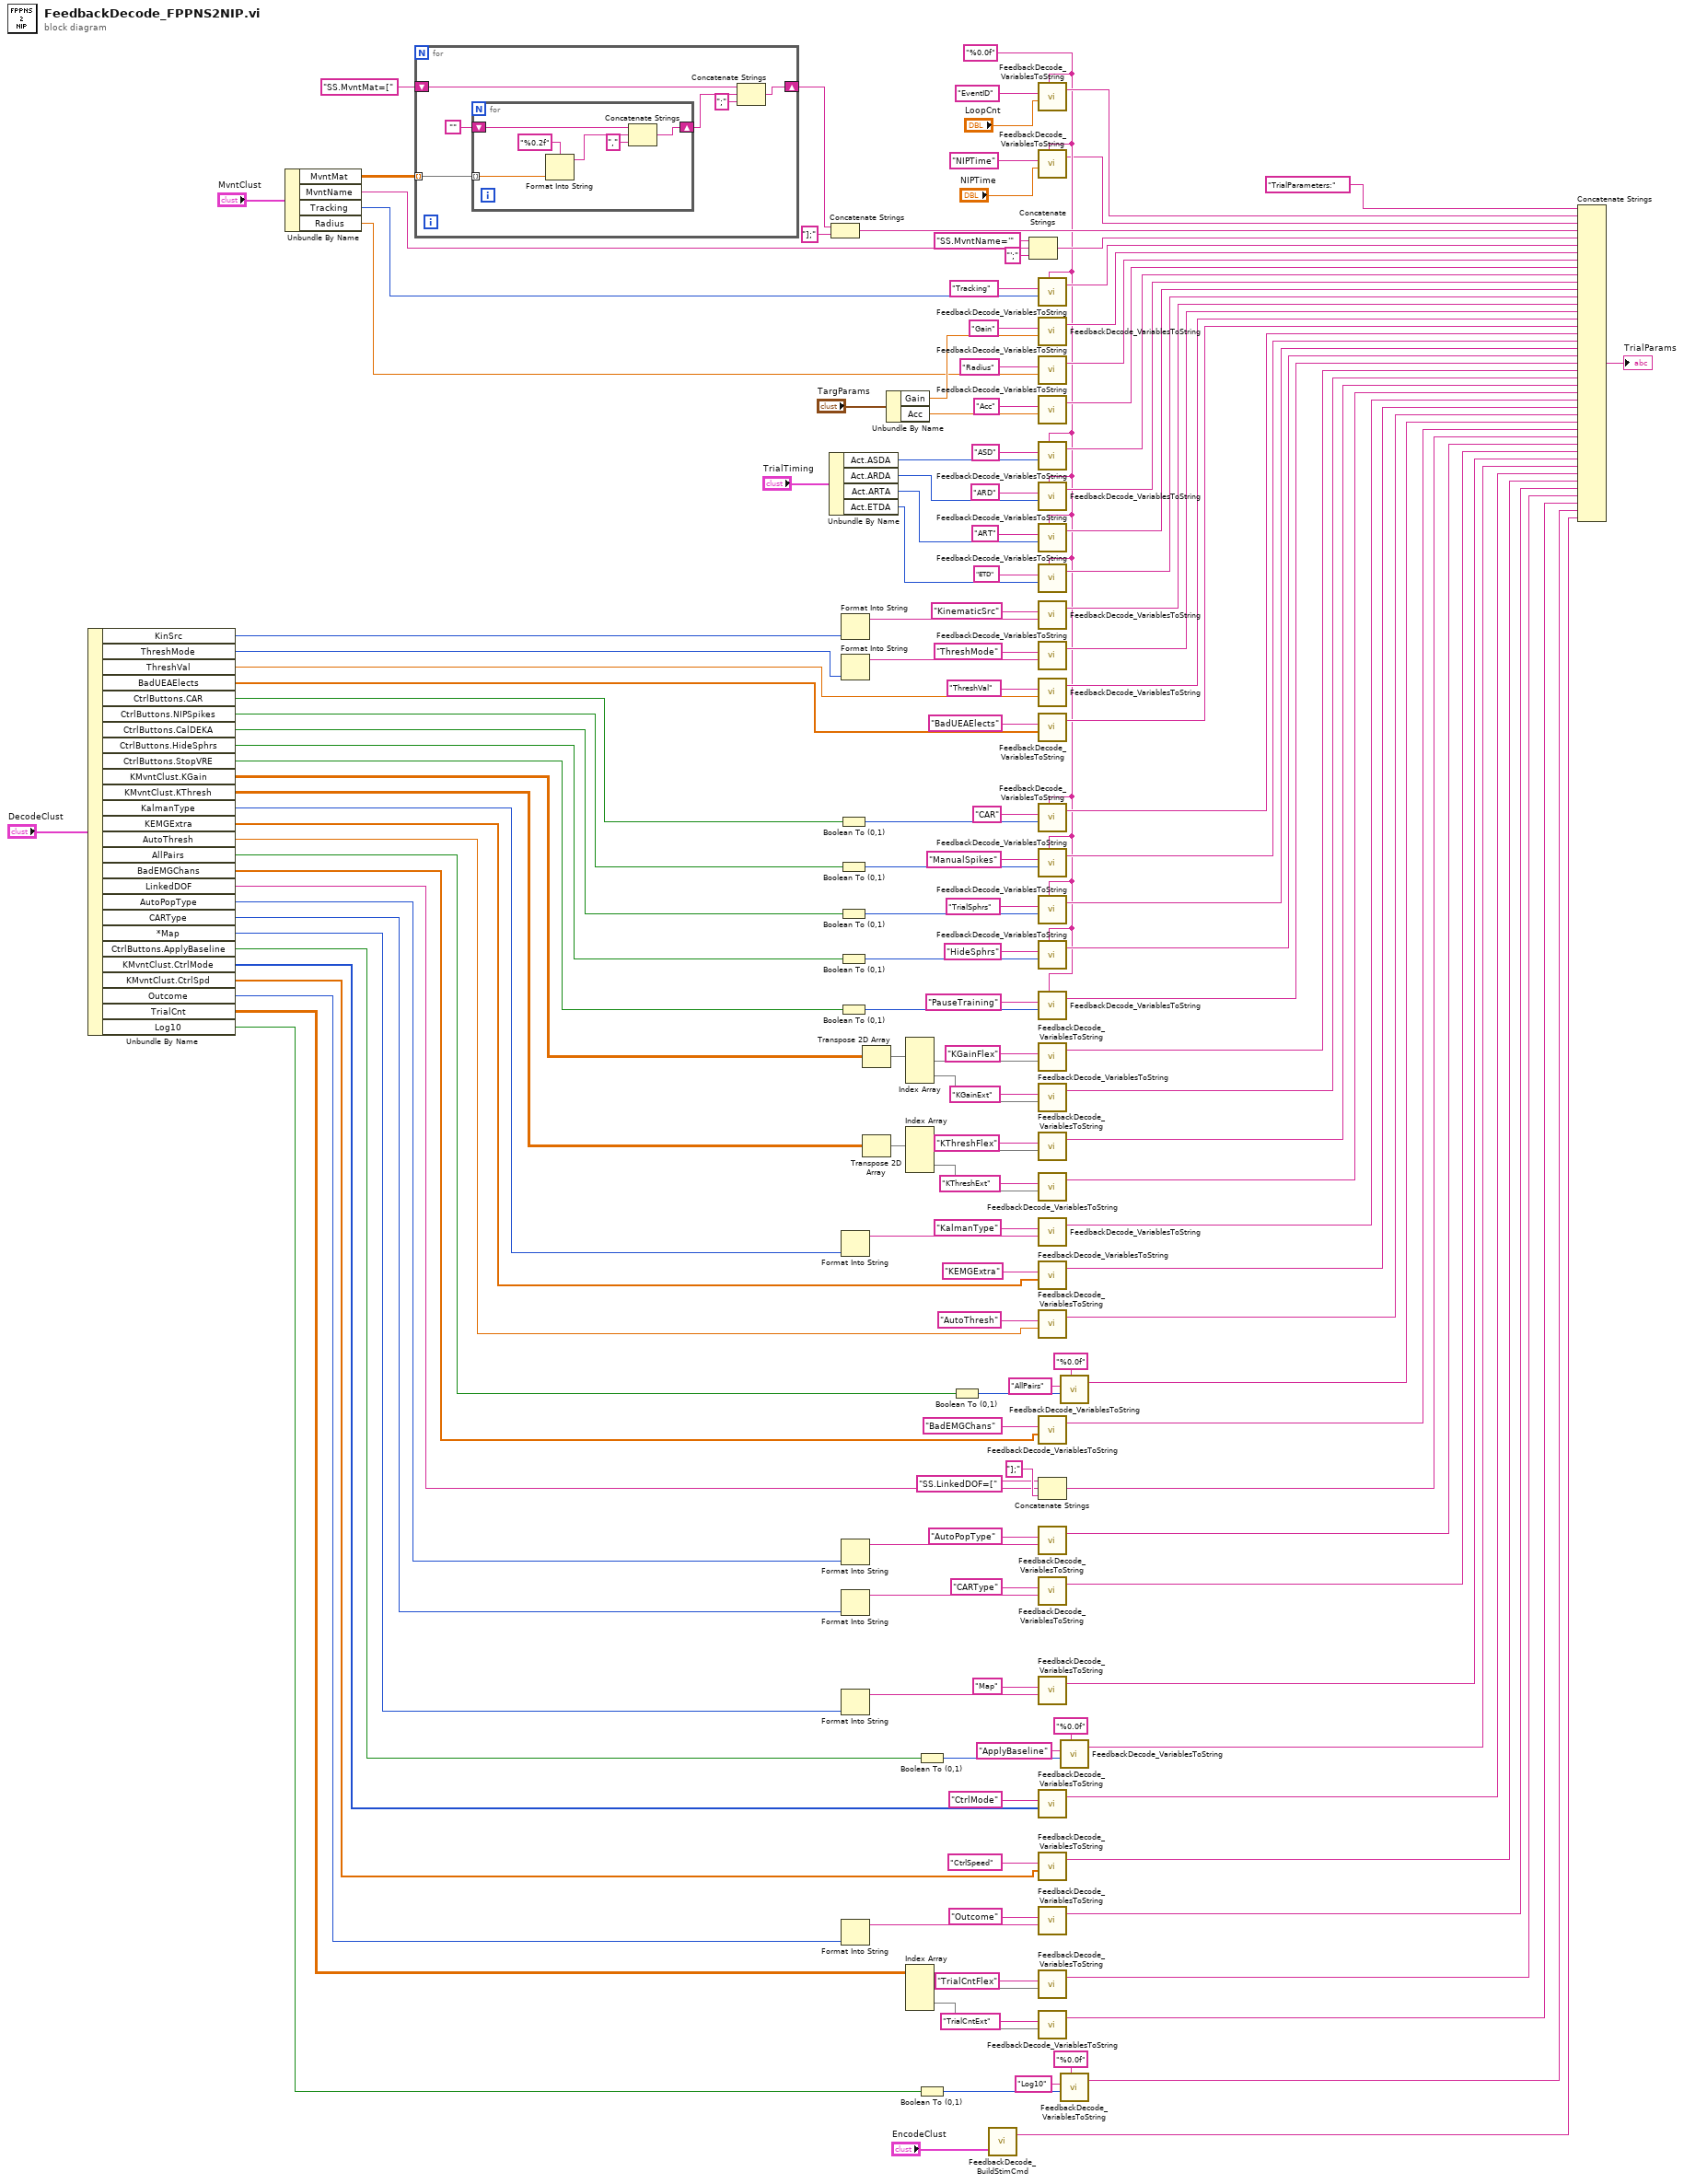
[diagram p0: block diagram]
diagram:
  w5 = "%0.0f" ("Format")
  n1 = Unbundle By Name("DecodeClust") -> ("KinSrc"=w116:T5, "ThreshMode"=w115:T6, "ThreshVal"=w113:dbl, "BadUEAElects"=w68:dbl[], "CtrlButtons.CAR"=w103:bool, "CtrlButtons.NIPSpikes"=w102:bool, "CtrlButtons.CalDEKA"=w101:bool, "CtrlButtons.HideSphrs"=w100:bool, "CtrlButtons.StopVRE"=w99:bool, "KMvntClust.KGain"=w82:sgl[][], "KMvntClust.KThresh"=w73:sgl[][], "KalmanType"=w79:T7, "KEMGExtra"=w65:dbl[], "AutoThresh"=w60:dbl, "AllPairs"=w59:bool, "BadEMGChans"=w54:dbl[], "LinkedDOF"=w46:string, "AutoPopType"=w45:enum16{"Standard", "Stepwise", "Gram"}, "CARType"=w44:enum16{"Standard", "NN"}, "*Map"=w38:T8, "CtrlButtons.ApplyBaseline"=w33:bool, "KMvntClust.CtrlMode"=w3:T9, "KMvntClust.CtrlSpd"=w28:sgl[], "Outcome"=w21:enum16{"---", "Success", "Failure"}, "TrialCnt"=w15:dbl[][], "Log10"=w9:bool)
  n2 = Unbundle By Name("MvntClust") -> ("MvntMat"=w125:dbl[][], "MvntName"=w121:string, "Tracking"=w118:enum8{"False", "True", "Mixed"}, "Radius"=w1:dbl)
  n3 = for {
    tunnel: w125 -> [w165] mode=indexing
    shift-right: [w160] -> w127
    shift-left: "SS.MvntMat=[" -> [w163]
    n4 = for {
      tunnel: w165 -> [w171] mode=indexing
      shift-right: [w166] -> w162
      shift-left: "" -> [w169]
      n5 = Format Into String(format string="%0.2f", w171) -> (resulting string=w168:string)  [unwired: 2 in, 1 out]
      n6 = Concatenate Strings(w169, w168, "," ("string")) -> (w166:string)
    }
    n7 = Concatenate Strings(w163, w162, ";" ("string")) -> (w160:string)
  }
  n8 = Unbundle By Name("TrialTiming") -> ("Act.ASDA"=w156:u16, "Act.ARDA"=w157:u16, "Act.ARTA"=w154:u16, "Act.ETDA"=w129:u16)
  n9 = Concatenate Strings(w127, "];" ("string")) -> (w124:string)
  n10 = Boolean To (0,1)(Boolean=w103) -> (0, 1=w147:i16)
  n11 = Boolean To (0,1)(Boolean=w102) -> (0, 1=w111:i16)
  n12 = Boolean To (0,1)(Boolean=w101) -> (0, 1=w108:i16)
  n13 = Boolean To (0,1)(Boolean=w100) -> (0, 1=w107:i16)
  n14 = Boolean To (0,1)(Boolean=w99) -> (0, 1=w104:i16)
  n15 = Format Into String(w116) -> (resulting string=w151:string)  [unwired: 3 in, 1 out]
  n16 = Format Into String(w115) -> (resulting string=w150:string)  [unwired: 3 in, 1 out]
  n17 = Format Into String(w79) -> (resulting string=w90:string)  [unwired: 3 in, 1 out]
  n18 = Format Into String(w45) -> (resulting string=w49:string)  [unwired: 3 in, 1 out]
  n19 = Format Into String(w44) -> (resulting string=w48:string)  [unwired: 3 in, 1 out]
  n20 = Format Into String(w38) -> (resulting string=w39:string)  [unwired: 3 in, 1 out]
  n21 = Format Into String(w21) -> (resulting string=w22:string)  [unwired: 3 in, 1 out]
  n22 = Transpose 2D Array(2D array=w82) -> (transposed array=w85:sgl[][])
  n23 = Transpose 2D Array(2D array=w73) -> (transposed array=w76:sgl[][])
  n24 = Unbundle By Name("TargParams") -> ("Gain"=w138:dbl, "Acc"=w137:dbl)
  n25 = Index Array(array=w85) -> (element #1=w86:sgl[], element #2=w87:sgl[])  [unwired: 4 in]
  n26 = Index Array(array=w76) -> (element #1=w75:sgl[], element #2=w74:sgl[])  [unwired: 4 in]
  n27 = Index Array(array=w15) -> (element #1=w18:dbl[], element #2=w19:dbl[])  [unwired: 4 in]
  n28 = Boolean To (0,1)(Boolean=w33) -> (0, 1=w34:i16)
  n29 = Boolean To (0,1)(Boolean=w9) -> (0, 1=w12:i16)
  n30 = Boolean To (0,1)(Boolean=w59) -> (0, 1=w63:i16)
  n31 = call "FeedbackDecode_BuildStimCmd.vi"("EncodeClustIn"="EncodeClust") -> ("StimCmd"=w24:string)  [unwired: 1 in, 1 out]
  n32 = Concatenate Strings("SS.MvntName='" ("string"), w121, "';" ("string")) -> (w119:string)
  n33 = call-poly "FeedbackDecode_VariablesToString.vi"("Format"=w5, "ValueIn"="LoopCnt", "FieldName"="EventID" ("Key Word")) -> ("StringOut"=w91:string)  [unwired: 4 in]
  n34 = call-poly "FeedbackDecode_VariablesToString.vi"("Format"=w5, "ValueIn"="NIPTime", "FieldName"="NIPTime" ("Key Word")) -> ("StringOut"=w4:string)  [unwired: 4 in]
  n35 = call-poly "FeedbackDecode_VariablesToString.vi"("Format"=w5, "ValueIn"=w118, "FieldName"="Tracking" ("Key Word")) -> ("StringOut"=w117:string)  [unwired: 4 in]
  n36 = call-poly "FeedbackDecode_VariablesToString.vi"("ValueIn"=w138, "FieldName"="Gain" ("Key Word")) -> ("StringOut"=w134:string)  [unwired: 5 in]
  n37 = call-poly "FeedbackDecode_VariablesToString.vi"("ValueIn"=w1, "FieldName"="Radius" ("Key Word")) -> ("StringOut"=w135:string)  [unwired: 5 in]
  n38 = call-poly "FeedbackDecode_VariablesToString.vi"("ValueIn"=w137, "FieldName"="Acc" ("Key Word")) -> ("StringOut"=w136:string)  [unwired: 5 in]
  n39 = call-poly "FeedbackDecode_VariablesToString.vi"("Format"=w5, "ValueIn"=w156, "FieldName"="ASD" ("Key Word")) -> ("StringOut"=w146:string)  [unwired: 4 in]
  n40 = call-poly "FeedbackDecode_VariablesToString.vi"("Format"=w5, "ValueIn"=w157, "FieldName"="ARD" ("Key Word")) -> ("StringOut"=w145:string)  [unwired: 4 in]
  n41 = call-poly "FeedbackDecode_VariablesToString.vi"("Format"=w5, "ValueIn"=w154, "FieldName"="ART" ("Key Word")) -> ("StringOut"=w144:string)  [unwired: 4 in]
  n42 = call-poly "FeedbackDecode_VariablesToString.vi"("Format"=w5, "ValueIn"=w129, "FieldName"="ETD" ("Key Word")) -> ("StringOut"=w98:string)  [unwired: 4 in]
  n43 = call-poly "FeedbackDecode_VariablesToString.vi"("ValueIn"=w151, "FieldName"="KinematicSrc" ("Key Word")) -> ("StringOut"=w143:string)  [unwired: 5 in]
  n44 = call-poly "FeedbackDecode_VariablesToString.vi"("ValueIn"=w150, "FieldName"="ThreshMode" ("Key Word")) -> ("StringOut"=w142:string)  [unwired: 5 in]
  n45 = call-poly "FeedbackDecode_VariablesToString.vi"("ValueIn"=w113, "FieldName"="ThreshVal" ("Key Word")) -> ("StringOut"=w112:string)  [unwired: 5 in]
  n46 = call-poly "FeedbackDecode_VariablesToString.vi"("ValueIn"=w68, "FieldName"="BadUEAElects" ("Key Word")) -> ("StringOut"=w67:string)  [unwired: 5 in]
  n47 = call-poly "FeedbackDecode_VariablesToString.vi"("Format"=w5, "ValueIn"=w147, "FieldName"="CAR" ("Key Word")) -> ("StringOut"=w141:string)  [unwired: 4 in]
  n48 = call-poly "FeedbackDecode_VariablesToString.vi"("Format"=w5, "ValueIn"=w111, "FieldName"="ManualSpikes" ("Key Word")) -> ("StringOut"=w97:string)  [unwired: 4 in]
  n49 = call-poly "FeedbackDecode_VariablesToString.vi"("Format"=w5, "ValueIn"=w108, "FieldName"="TrialSphrs" ("Key Word")) -> ("StringOut"=w96:string)  [unwired: 4 in]
  n50 = call-poly "FeedbackDecode_VariablesToString.vi"("Format"=w5, "ValueIn"=w107, "FieldName"="HideSphrs" ("Key Word")) -> ("StringOut"=w95:string)  [unwired: 4 in]
  n51 = call-poly "FeedbackDecode_VariablesToString.vi"("Format"=w5, "ValueIn"=w104, "FieldName"="PauseTraining" ("Key Word")) -> ("StringOut"=w94:string)  [unwired: 4 in]
  n52 = call-poly "FeedbackDecode_VariablesToString.vi"("ValueIn"=w86, "FieldName"="KGainFlex" ("Key Word")) -> ("StringOut"=w81:string)  [unwired: 5 in]
  n53 = call-poly "FeedbackDecode_VariablesToString.vi"("ValueIn"=w87, "FieldName"="KGainExt" ("Key Word")) -> ("StringOut"=w80:string)  [unwired: 5 in]
  n54 = call-poly "FeedbackDecode_VariablesToString.vi"("ValueIn"=w75, "FieldName"="KThreshFlex" ("Key Word")) -> ("StringOut"=w72:string)  [unwired: 5 in]
  n55 = call-poly "FeedbackDecode_VariablesToString.vi"("ValueIn"=w74, "FieldName"="KThreshExt" ("Key Word")) -> ("StringOut"=w71:string)  [unwired: 5 in]
  n56 = call-poly "FeedbackDecode_VariablesToString.vi"("ValueIn"=w90, "FieldName"="KalmanType" ("Key Word")) -> ("StringOut"=w88:string)  [unwired: 5 in]
  n57 = call-poly "FeedbackDecode_VariablesToString.vi"("ValueIn"=w65, "FieldName"="KEMGExtra" ("Key Word")) -> ("StringOut"=w58:string)  [unwired: 5 in]
  n58 = call-poly "FeedbackDecode_VariablesToString.vi"("ValueIn"=w60, "FieldName"="AutoThresh" ("Key Word")) -> ("StringOut"=w57:string)  [unwired: 5 in]
  n59 = call-poly "FeedbackDecode_VariablesToString.vi"("ValueIn"=w54, "FieldName"="BadEMGChans" ("Key Word")) -> ("StringOut"=w53:string)  [unwired: 5 in]
  n60 = Concatenate Strings("SS.LinkedDOF=[" ("Key Word"), w46, "];" ("string")) -> (w43:string)
  n61 = call-poly "FeedbackDecode_VariablesToString.vi"("ValueIn"=w49, "FieldName"="AutoPopType" ("Key Word")) -> ("StringOut"=w42:string)  [unwired: 5 in]
  n62 = call-poly "FeedbackDecode_VariablesToString.vi"("ValueIn"=w48, "FieldName"="CARType" ("Key Word")) -> ("StringOut"=w41:string)  [unwired: 5 in]
  n63 = call-poly "FeedbackDecode_VariablesToString.vi"("ValueIn"=w39, "FieldName"="Map" ("Key Word")) -> ("StringOut"=w37:string)  [unwired: 5 in]
  n64 = call-poly "FeedbackDecode_VariablesToString.vi"("ValueIn"=w3, "FieldName"="CtrlMode" ("Key Word")) -> ("StringOut"=w30:string)  [unwired: 5 in]
  n65 = call-poly "FeedbackDecode_VariablesToString.vi"("ValueIn"=w28, "FieldName"="CtrlSpeed" ("Key Word")) -> ("StringOut"=w27:string)  [unwired: 5 in]
  n66 = call-poly "FeedbackDecode_VariablesToString.vi"("ValueIn"=w22, "FieldName"="Outcome" ("Key Word")) -> ("StringOut"=w20:string)  [unwired: 5 in]
  n67 = call-poly "FeedbackDecode_VariablesToString.vi"("ValueIn"=w18, "FieldName"="TrialCntFlex" ("Key Word")) -> ("StringOut"=w14:string)  [unwired: 5 in]
  n68 = call-poly "FeedbackDecode_VariablesToString.vi"("ValueIn"=w19, "FieldName"="TrialCntExt" ("Key Word")) -> ("StringOut"=w13:string)  [unwired: 5 in]
  n69 = call-poly "FeedbackDecode_VariablesToString.vi"("Format"="%0.0f", "ValueIn"=w63, "FieldName"="AllPairs") -> ("StringOut"=w56:string)  [unwired: 4 in]
  n70 = call-poly "FeedbackDecode_VariablesToString.vi"("Format"="%0.0f", "ValueIn"=w34, "FieldName"="ApplyBaseline") -> ("StringOut"=w32:string)  [unwired: 4 in]
  n71 = call-poly "FeedbackDecode_VariablesToString.vi"("Format"="%0.0f", "ValueIn"=w12, "FieldName"="Log10") -> ("StringOut"=w8:string)  [unwired: 4 in]
  n72 = Concatenate Strings("TrialParameters:" ("string"), w91, w4, w124, w119, w117, w134, w135, w136, w146, w145, w144, w98, w143, w142, w112, w67, w141, w97, w96, w95, w94, w81, w80, w72, w71, w88, w58, w57, w56, w53, w43, w42, w41, w37, w32, w30, w27, w20, w14, w13, w8, w24) -> (→"TrialParams":string)
